vi "Get Sweep Pattern Subset.vi"(6 "Sampling":cluster{"Fs":dbl, "#s":i32}, 8 "error in (no error)":errorcluster, 10 "index":i32, 11 "Sweep Pattern":dbl[](array[numeric])) -> (0 "error out":errorcluster, 2 "Pattern Subset":dbl[](array[numeric]), 3 "output waveform":waveform(dbl))   [LabVIEW 2016, in "Lockin.DAQ.lvclass"]
uses:
  Lockin.DAQ.lvclass
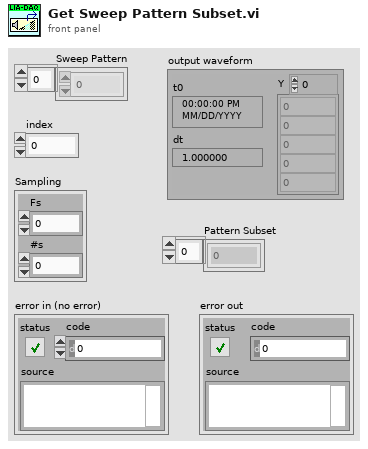
[diagram p1: front panel]
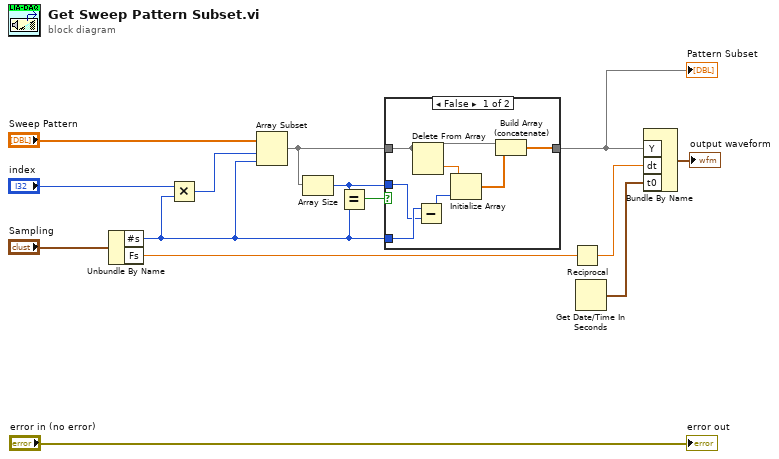
[diagram p0: block diagram]
diagram:
  n1 = Unbundle By Name("Sampling") -> ("#s"=w5:i32, "Fs"=w6:dbl)
  n2 = Multiply(x="index", y=w5) -> (x*y=w10:i32)
  n3 = Array Subset(array="Sweep Pattern", index=w10, length=w5) -> (w2:dbl[])
  n4 = Array Size(array=w2) -> (size(s)=w4:i32)
  n5 = Equal?(x=w4, y=w5) -> (x = y?=w3:bool)
  n6 = case shown="False" w3 {
    tunnel: w5 -> [w21 _]
    tunnel: w4 -> [w20 _]
    tunnel: w2 -> [w16 w22]
    tunnel: [w15 w22] -> w1
    frame False {
      n7 = Delete From Array(array=w16) -> (deleted portion=w18:dbl)  [unwired: 2 in, 1 out]
      n8 = Subtract(x=w21, y=w20) -> (x-y=w19:i32)
      n9 = Initialize Array(w18, w19) -> (w17:dbl[])
      n10 = Build Array (concatenate)(w16, w17) -> (w15:dbl[])
    }
    frame True {
    }
  }
  "Pattern Subset" <- w1
  n11 = Reciprocal(x=w6) -> (1/x=w8:dbl)
  n12 = Get Date/Time In Seconds() -> (seconds since 1Jan1904=w9:timestamp)
  n13 = Bundle By Name("Y"=w1, "dt"=w8, "t0"=w9) -> (→"output waveform":waveform(dbl))  [unwired: 1 in]
  "error out" <- "error in (no error)"
